vi "File.Fix Start of Network File Path.vi"(11 "String Path":string) -> (3 "String Path Out":string)   [LabVIEW 2018]
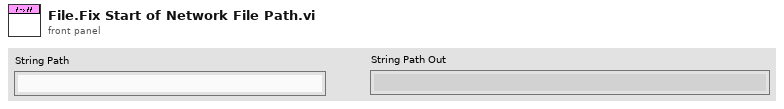
[diagram p1: front panel]
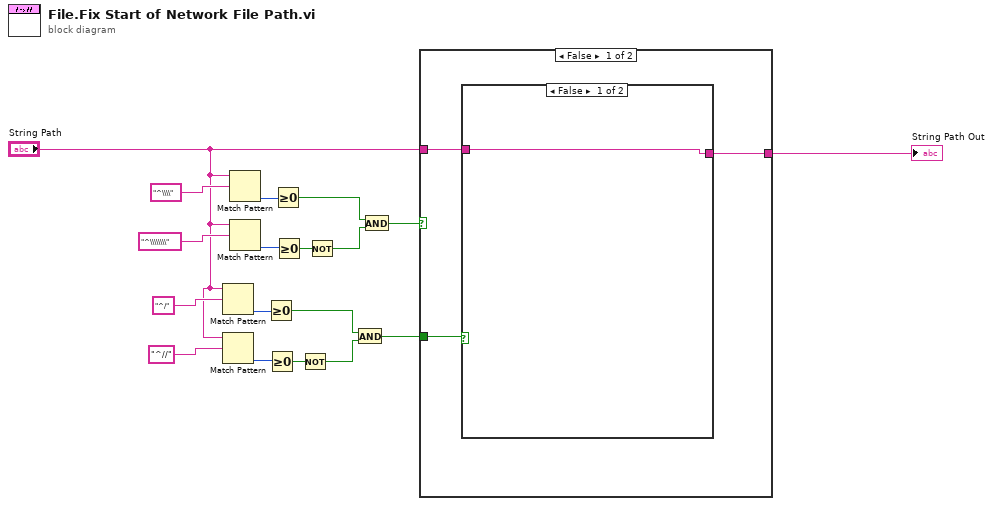
[diagram p0: block diagram]
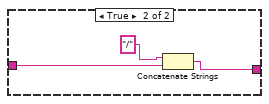
[diagram p2: hidden frame]
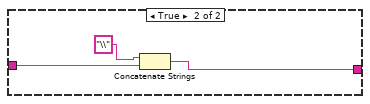
[diagram p3: hidden frame]
diagram:
  n1 = Match Pattern(string="String Path", regular expression="^/") -> (offset past match=w5:i32)  [unwired: 1 in, 3 out]
  n2 = Match Pattern(string="String Path", regular expression="^//") -> (offset past match=w6:i32)  [unwired: 1 in, 3 out]
  n3 = Match Pattern(string="String Path", regular expression="^\\\\") -> (offset past match=w16:i32)  [unwired: 1 in, 3 out]
  n4 = Match Pattern(string="String Path", regular expression="^\\\\\\\\") -> (offset past match=w15:i32)  [unwired: 1 in, 3 out]
  n5 = Greater Or Equal To 0?(x=w5) -> (x >= 0?=w9:bool)
  n6 = Greater Or Equal To 0?(x=w6) -> (x >= 0?=w7:bool)
  n7 = Greater Or Equal To 0?(x=w16) -> (x >= 0?=w12:bool)
  n8 = Greater Or Equal To 0?(x=w15) -> (x >= 0?=w14:bool)
  n9 = Not(x=w7) -> (.not. x?=w8:bool)
  n10 = Not(x=w14) -> (.not. x?=w13:bool)
  n11 = And(x=w9, y=w8) -> (x .and. y?=w1:bool)
  n12 = And(x=w12, y=w13) -> (x .and. y?=w10:bool)
  n13 = case shown="False" w10 {
    tunnel: "String Path" -> [w20 w28]
    tunnel: [w19 w27] -> w11
    tunnel: w1 -> [w21 _]
    frame False {
      n14 = case shown="False" w21 {
        tunnel: w20 -> [w22 w24]
        tunnel: [w22 w23] -> w19
        frame False {
        }
        frame True {
          n15 = Concatenate Strings("/" ("regular expression"), w24) -> (w23:string)
        }
      }
    }
    frame True {
      n16 = Concatenate Strings("\\" ("regular expression"), w28) -> (w27:string)
    }
  }
  "String Path Out" <- w11
